vi "GCFS.vi"() -> ()   [LabVIEW 2024]
uses:
  DataCluster_GCFS.ctl
  <vilib>/userDefined/High Color/IMAQdx.ctl
  <vilib>/vision/Image Controls.llb/IMAQ Image.ctl
  <vilib>/Platform/TimedLoop/XDataNode/timing_clust.ctl
  <vilib>/Platform/TimedLoop/XDataNode/nitl_modes.ctl
  <vilib>/Platform/TimedLoop/XDataNode/wakeup.ctl
  af9ea1de-6e94-45bd-9990-e3be68a33346.vi
  <vilib>/addons/_JKI Toolkits/State Machine/_JKI_lib_State_Machine.llb/Select State(s)_err__jki_lib_state_machine.vi
  <extravilib>/ChannelInstances/Tag-t'DataCluster_GCFS.ctl'/Read With Abort.vi
  <extravilib>/ChannelInstances/Stream-c(t'IMAQ Image.ctl',str,a[.,.](str),a[.,.](str),bool)/Read With Abort.vi
  <extravilib>/ChannelInstances/Stream-c(t'IMAQ Image.ctl',str,a[.,.](str),a[.,.](str),bool)/Write With Abort.vi
  <extravilib>/ChannelInstances/Tag-t'DataCluster_GCFS.ctl'/Write With Abort.vi
  <extravilib>/ChannelInstances/Stream-c(t'IMAQ Image.ctl',str,a[.,.](str),a[.,.](str),bool)/EndpointRead.vi
  <extravilib>/ChannelInstances/Stream-c(t'IMAQ Image.ctl',str,a[.,.](str),a[.,.](str),bool)/Endpoint.vi
  <extravilib>/ChannelInstances/Stream-c(t'IMAQ Image.ctl',str,a[.,.](str),a[.,.](str),bool)/Instantiate.vi
  <extravilib>/ChannelInstances/Tag-t'DataCluster_GCFS.ctl'/Instantiate.vi
  <extravilib>/ChannelInstances/Tag-t'DataCluster_GCFS.ctl'/EndpointRead.vi
  <extravilib>/ChannelInstances/Stream-c(t'IMAQ Image.ctl',str,a[.,.](str),a[.,.](str),bool)/)Channel.vi
  <resource>/ChannelSupport/_ChannelSupport/WaitIfNeeded.vi
  <vilib>/addons/_JKI Toolkits/State Machine/_JKI_lib_State_Machine.llb/Periodic Trigger__ogtk__JKI-SM__jki_lib_state_machine.vi
  <vilib>/Utility/file.llb/Write Delimited Spreadsheet (DBL).vi
  <extravilib>/ChannelInstances/Tag-t'DataCluster_GCFS.ctl'/Endpoint.vi
  <vilib>/platform/TimedLoop/XDataNode/XDataNode.xnode
  <vilib>/regexp/Match Regular Expression.xnode
  <vilib>/vision/driver/NI_Vision_Acquisition_Software.lvlib
  <extravilib>/ChannelInstances/Tag-t'DataCluster_GCFS.ctl'.lvlib
  <vilib>/Platform/TimedLoop/XDataNode/XDNodeRunTimeDep.lvlib
  <extravilib>/ChannelInstances/Stream-c(t'IMAQ Image.ctl',str,a[.,.](str),a[.,.](str),bool).lvlib
panel:
  in  "Use Test Image":bool
  out "Save loop":i32
  out "Data Loop":i32
  out "Temperature":dbl
  in  "Freezing value":sgl=250.0
  in  "OFF":bool
  in  "Cool":bool
  in  "Heat":bool
  in  "Get Image":bool
  out "Frezz Image":T1(plugin-control)
  out "Droplet binary":T1(plugin-control)
  out "Droplet Position":T1(plugin-control)
  out "Grap Image":T1(plugin-control)
  in  "Active":bool
  in  "Sample name":string
  in  "Grap Position Image":bool
  out "Statusstring":string
  out "Particle Measurements (Pixels) (Particle Analysis 1)":dbl[][](array[numeric]) format="%.2f"
  out "Number of Particles":i32
  in  "Exit":bool
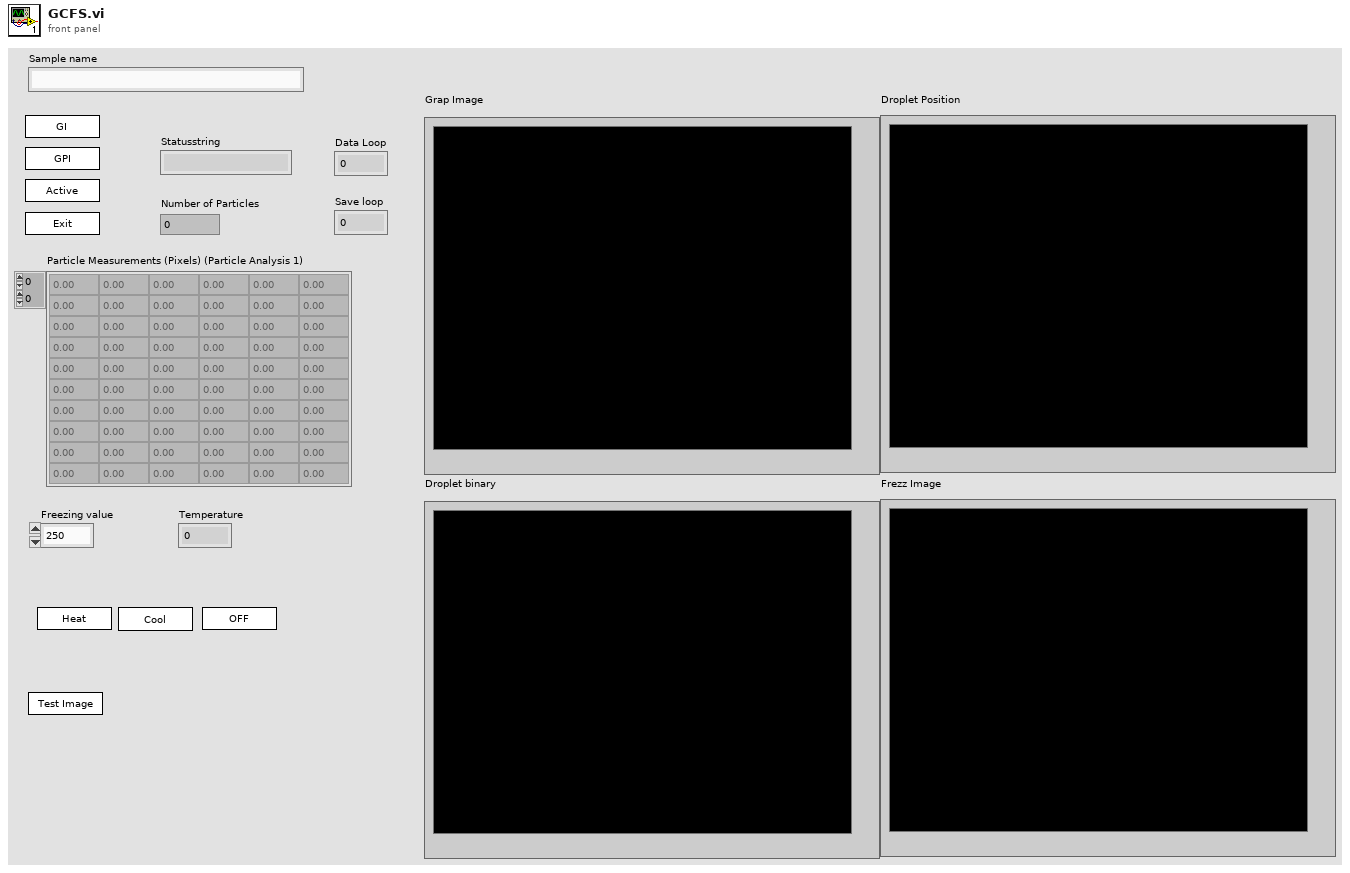
[diagram p1: front panel]
types:
  T1 = typedef "IMAQ Image.ctl" = refnum<image>
  T2 = typedef "DataCluster_GCFS.ctl" = cluster{"Core":cluster{"Current VI Reference":refnum<vi>, "Close Panel on Exit?":bool}, "Your Boolean data":bool, "Your string data":string, "Camera Cluster":cluster{"Session":T3, "Image":T1, "Position Image":T1, "PixelVal Image":T1, "Position Image Binary":T1, "Lable Image":T1}, "Data In Cluster":cluster{"Images":cluster{"Position Image path":path, "Sample folder path":path, "Label Image path":path}, "Sample Name":string, "Sample Rate":i32, "Gradient Buffer":i32, "Data Acquisition.Setup.TempGrad":dbl, "Control.PID gains":cluster{"proportional gain (Kc)":dbl, "integral time (Ti, min)":dbl, "derivative time (Td, min)":dbl}}, "Active":bool, "Ready":bool, "Exit":bool, "Arduino":cluster{"Connection":bool, "Port":refnum<visa-resource-name>, "State":string}, "Program_Start":string, "Data Out Cluster":cluster{"Particle Measurements (Pixels) (Particle Analysis 1)":dbl[][], "Number of droplets":i32, "PosImg_Timestamp":string}, "PSU":cluster{"Connection":bool, "Port":refnum<visa-resource-name>, "State":string}}
  T3 = typedef "IMAQdx.ctl" = refnum<k21>
  T4 = enum32{"Invalid", "Standard", "Closed", "Hidden", "Minimized", "Maximized"}
  T5 = enum32{"invalid app kind", "Development System", "Run Time System", "Student Edition", "Embedded LabVIEW", "Evaluation", "Custom"}
  T6 = cluster{"Desired Font (Application)":enum16{"User-specified Font", "Application Font", "System Font", "Dialog Font"}, "[User-specified Font]":cluster{"Font Name":string, "Size":i16, "Strikeout?":bool, "Italic?":bool, "Underline?":bool, "Outline?":bool, "Shadow?":bool, "Bold?":bool, "Rotation Angle":dbl}, "Horizontal Alignment":i16, "Vertical Alignment":i16}
  T7 = cluster{"Current VI Reference":refnum<vi>, "Close Panel on Exit?":bool}
  T8 = typedef "Image Type" = u32
  T9 = cluster{"Type":u32, "Version":u32, "Flags":u32, "SerialNumberHigh":u32, "SerialNumberLow":u32, "BusType":u32, "InterfaceName":string, "VendorName":string, "ModelName":string, "CameraFileName":string, "CameraAttributeURL":string}[]
  T10 = typedef "Tag-t'DataCluster_GCFS.ctl'.lvlib/))Channel.ctl" = refnum<queue>
  T11 = cluster{"Image To Save":T1, "Snap timestamp":string, "Pixel values":string[][], "Freezing points":string[][], "FreezingData":bool}
  T12 = typedef "XDNodeRunTimeDep.lvlib/timing_clust.ctl" = cluster{"Expected End [f-1]":u64, "Actual End [f-1]":u64, "Finished Late? [f-1]":bool, "Expected End [i-1]":u64, "Actual End [i-1]":u64, "Finished Late? [i-1]":bool, "Expected Start [i]":u64, "Actual Start [i]":u64, "Expected Start [f]":u64, "Actual Start [f]":u64, "Source Name":string, "Structure Name":string, "Period":i64, "Deadline":i64, "Offset":i64, "Start":i64, "Priority":i32, "Timeout":i32, "Mode":T13, "Wakeup Reason":T14, "Error":errorcluster, "Source Type":string, "Secondary Source Type":string, "Global End Time":u64, "Global Start Time":u64, "Frame Duration":u64, "Iteration Duration":u64, "Assigned CPU":i32, "I/O Scan Engine Mode":u32}
  T13 = typedef "XDNodeRunTimeDep.lvlib/nitl_modes.ctl" = enum32{"No Change", "Process missed periods, maintain original phase", "Discard missed periods, maintain original phase", "Process missed periods, ignore original phase", "Discard missed periods, ignore original phase"}
  T14 = typedef "XDNodeRunTimeDep.lvlib/wakeup.ctl" = enum32{"Normal", "Aborted", "Asynchronous wakeup", "Timing source error", "Timed loop error", "Timeout"}
  T15 = typedef "Stream-c(t'IMAQ Image.ctl',str,a[.,.](str),a[.,.](str),bool).lvlib/)Channel.ctl" = refnum<queue>
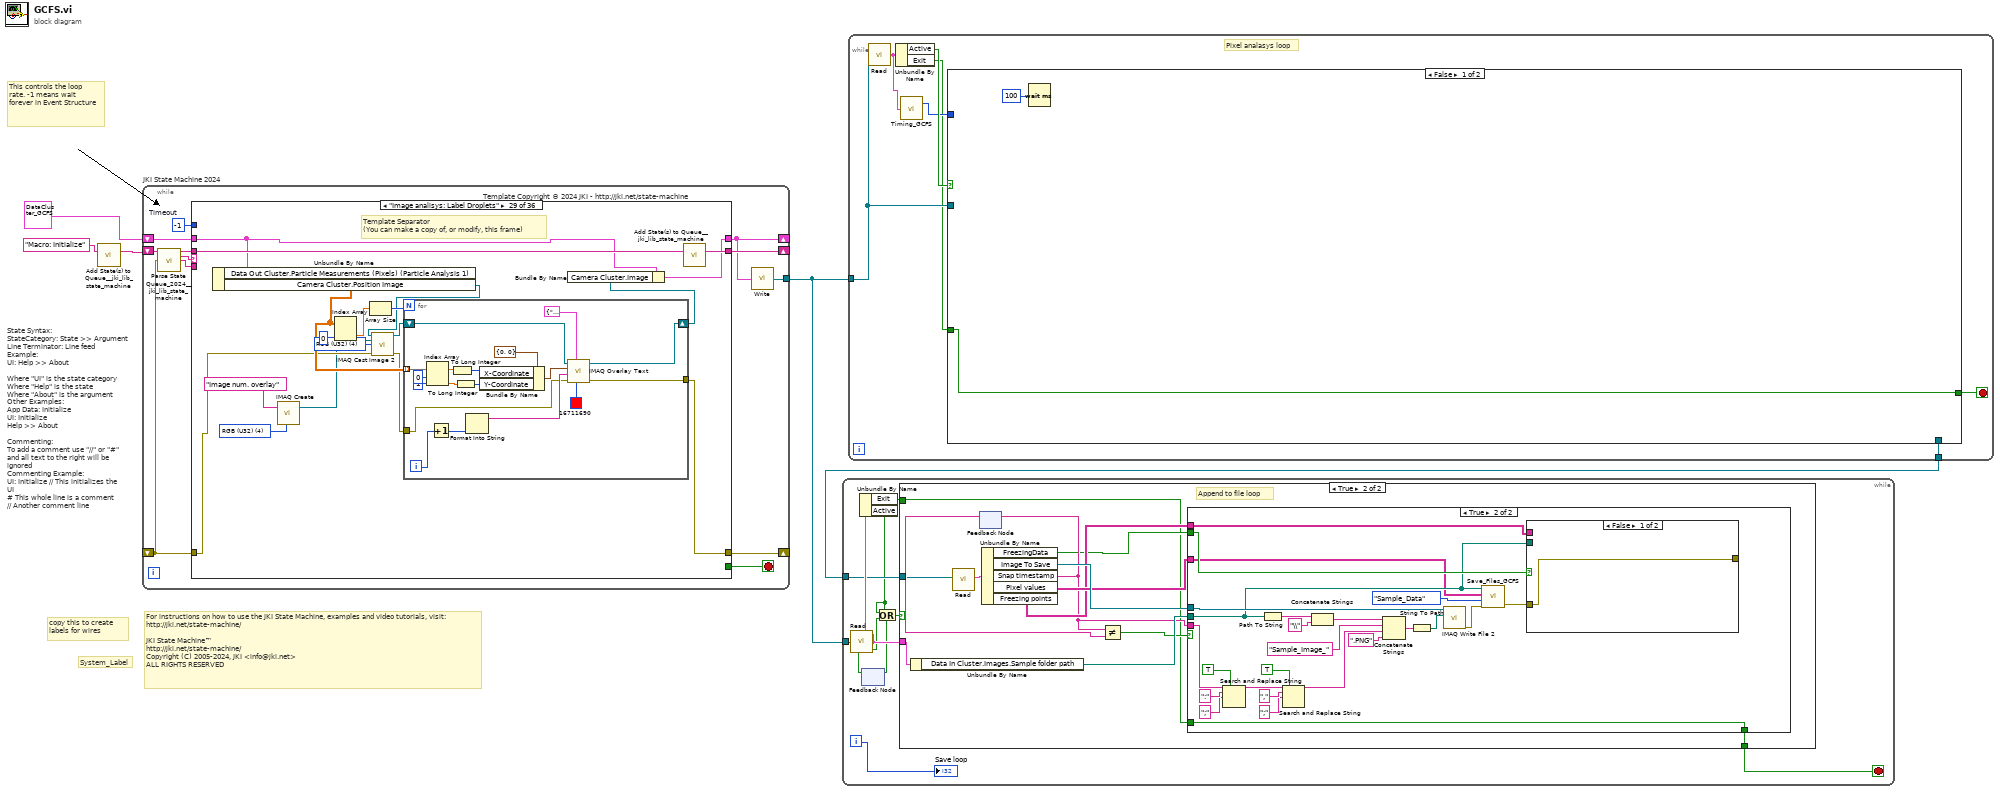
[diagram p0: block diagram]
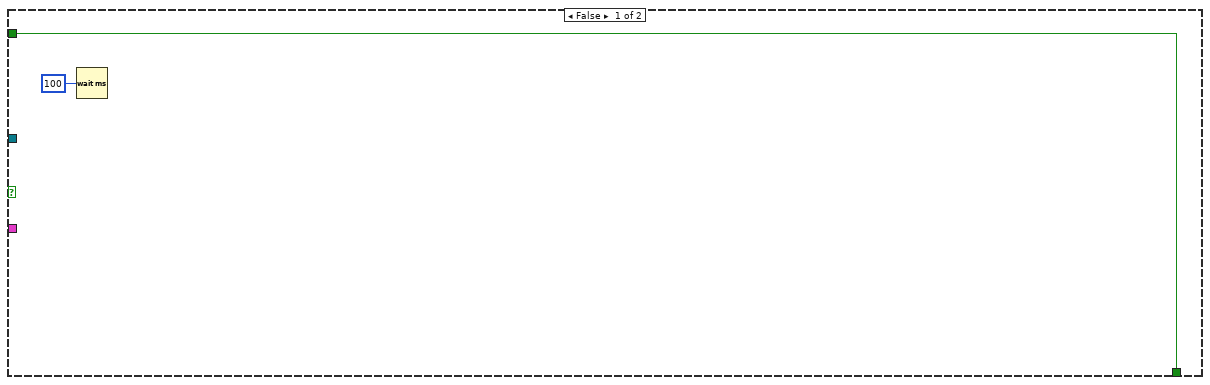
[diagram p2: hidden frame]
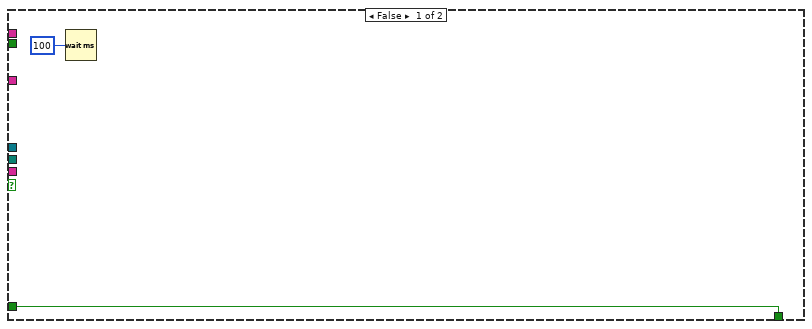
[diagram p3: hidden frame]
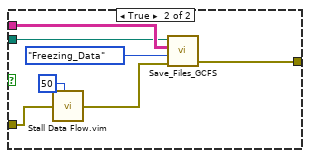
[diagram p4: hidden frame]
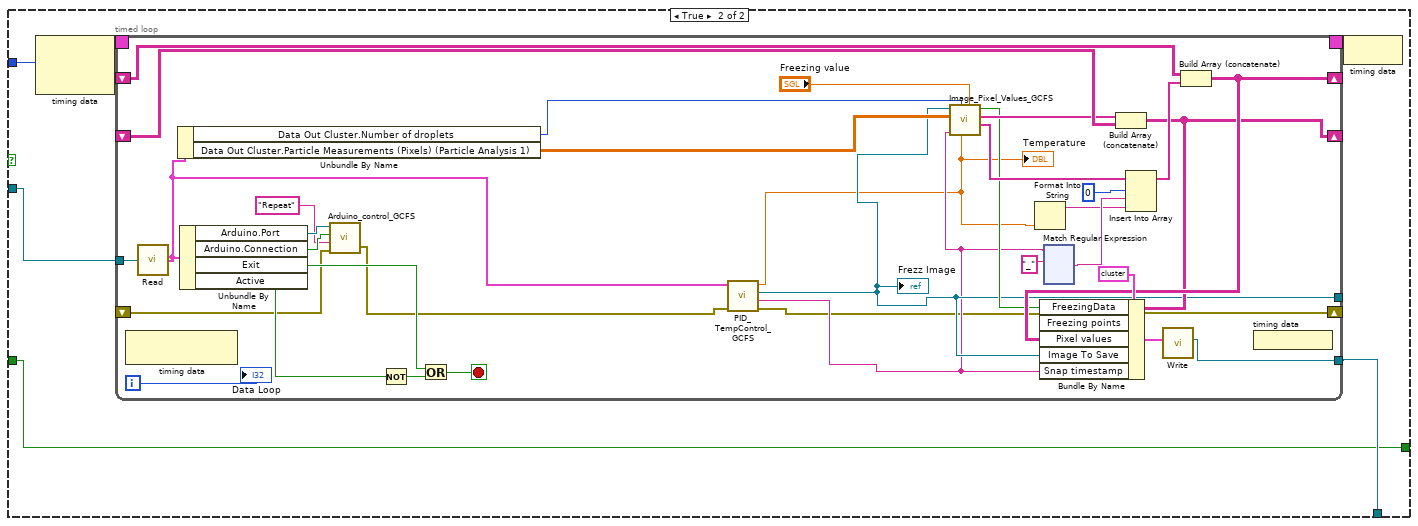
[diagram p5: hidden frame]
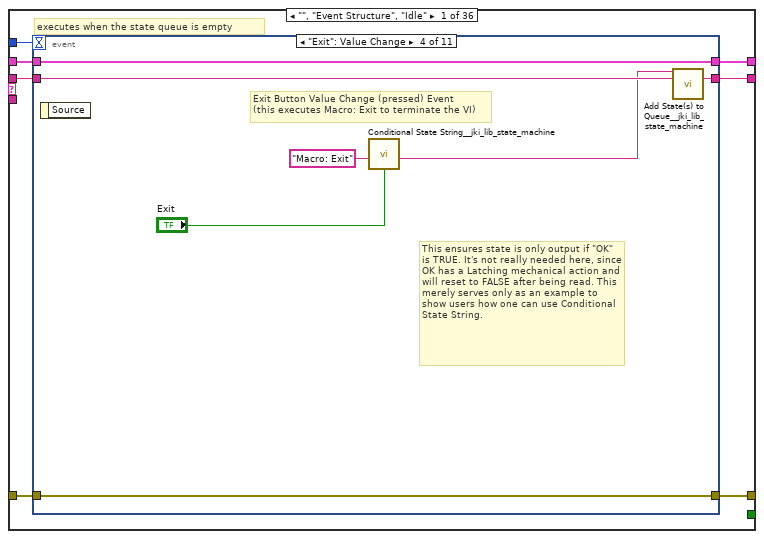
[diagram p6: hidden frame]
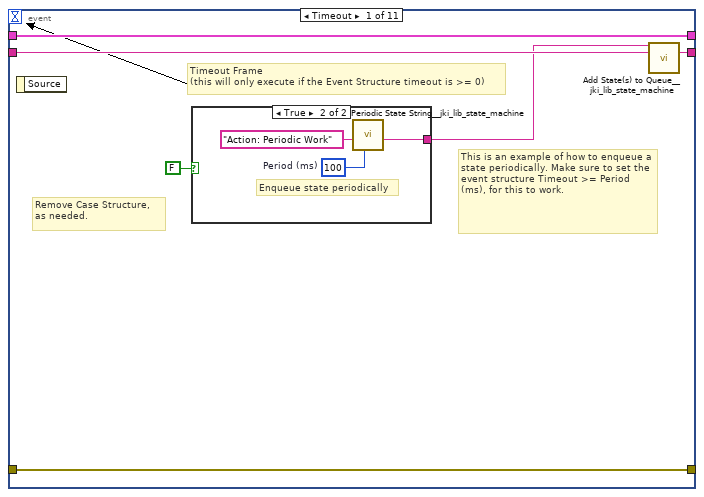
[diagram p7: hidden frame]
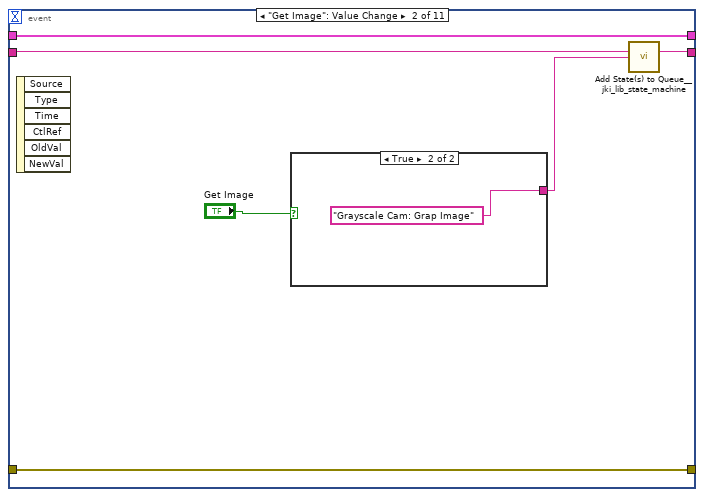
[diagram p9: hidden frame]
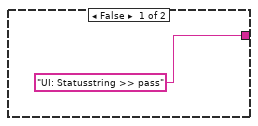
[diagram p10: hidden frame]
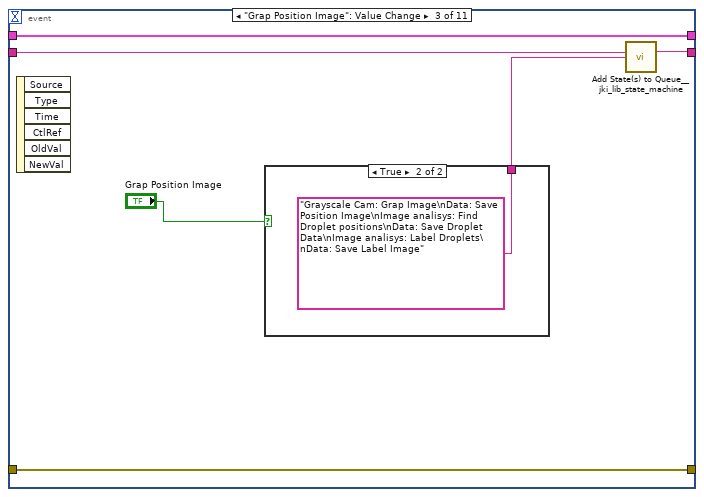
[diagram p11: hidden frame]
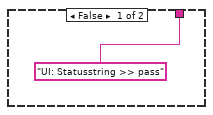
[diagram p12: hidden frame]
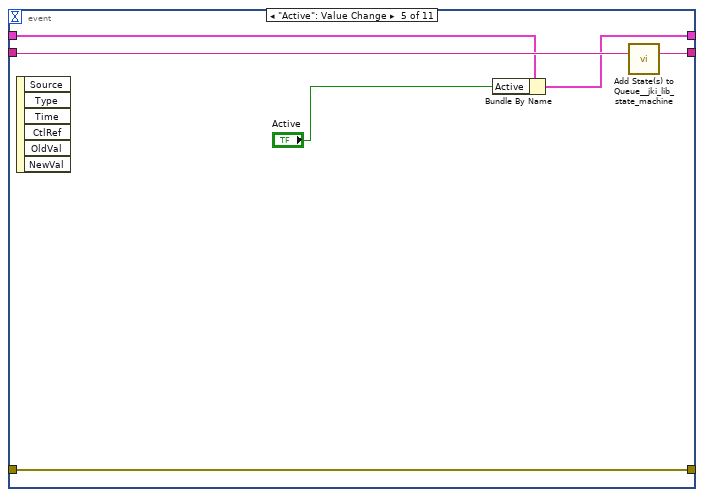
[diagram p13: hidden frame]
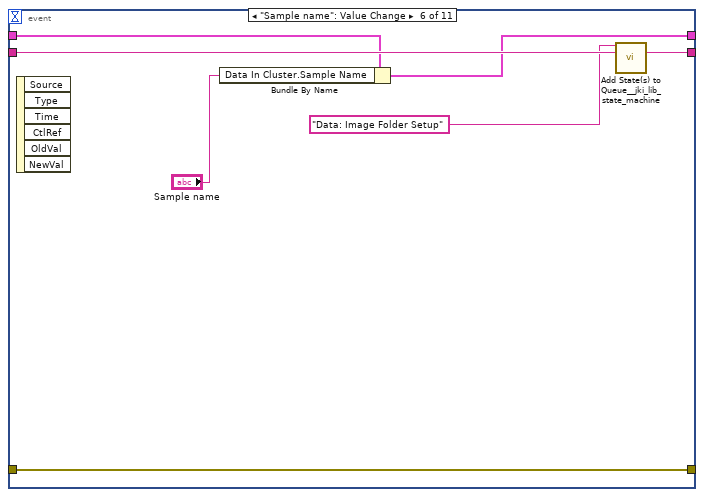
[diagram p14: hidden frame]
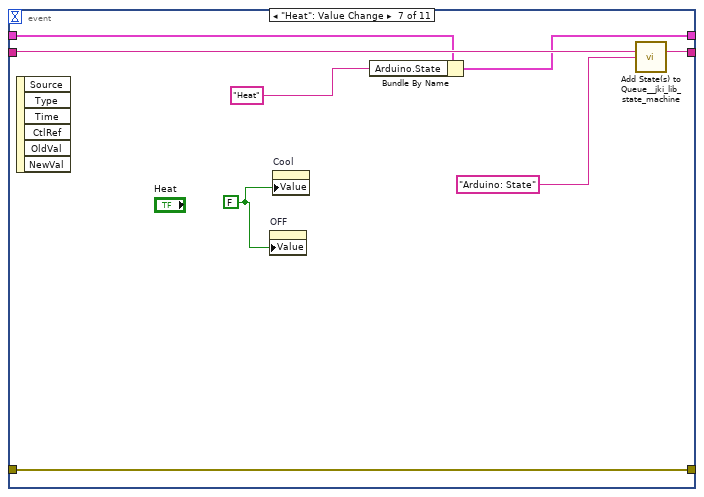
[diagram p15: hidden frame]
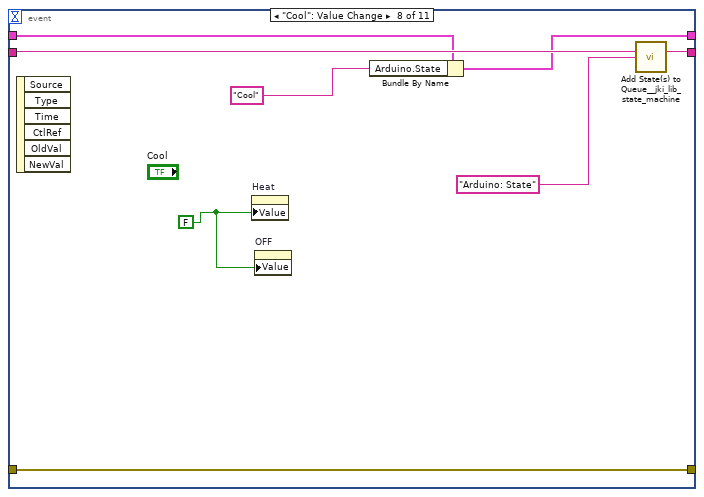
[diagram p16: hidden frame]
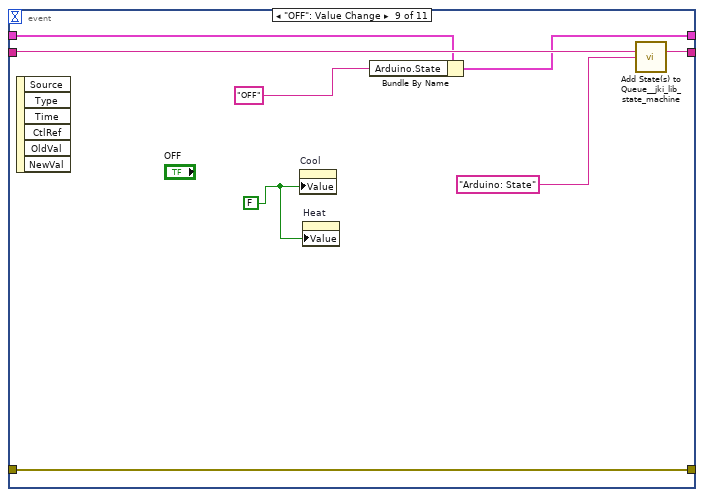
[diagram p17: hidden frame]
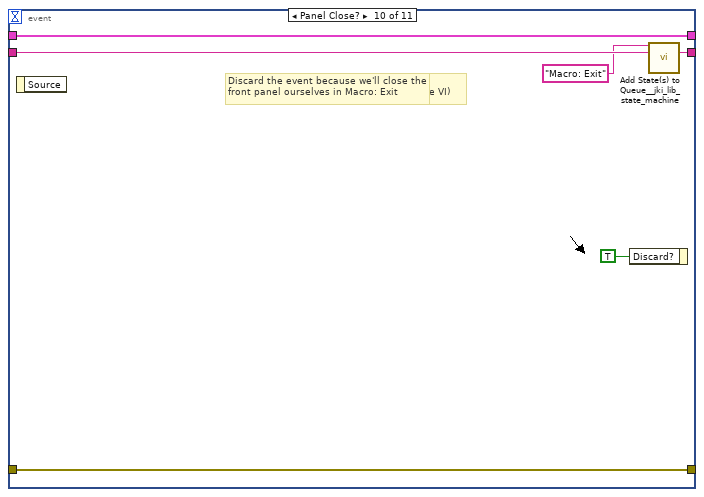
[diagram p18: hidden frame]
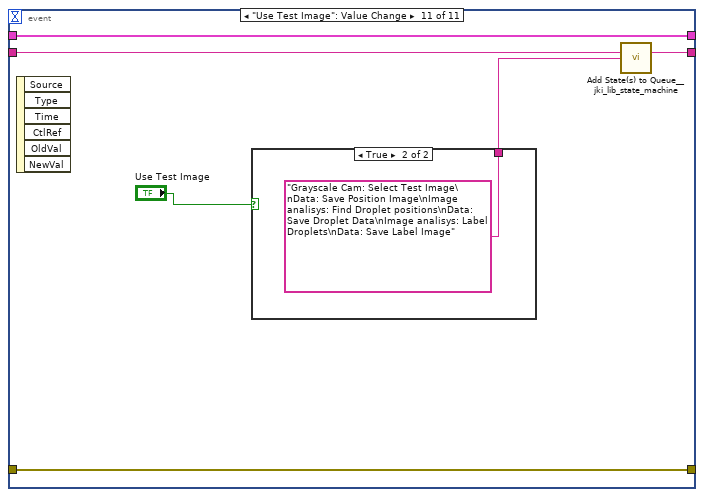
[diagram p19: hidden frame]
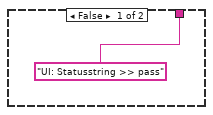
[diagram p20: hidden frame]
diagram:
  # "For instructions on how to use the JKI State Machine, examples and video tutorials, visit:\nhttp://jki.net/state-machine/\n\nJKI State Machine™\nhttp://jki.net/state-machine/\nCopyright (C) 2005-2024, JKI <info@jki.net>\nALL RIGHTS RESERVED"
  # "State Syntax:\nStateCategory: State >> Argument\nLine Terminator: Line feed\nExample:\nUI: Help >> About\n\nWhere \"UI\" is the state category\nWhere \"Help\" is the state\nWhere \"About\" is the argument\nOther Examples:\nApp Data: Initialize\nUI: Initialize\nHelp >> About\n\nCommenting:\nTo add a comment use \"//\" or \"#\" and all text to the right will be ignored\nCommenting Example:\nUI: Initialize // This initializes the UI\n# This whole line is a comment\n// Another comment line"
  # "copy this to create labels for wires"
  # "This controls the loop rate. -1 means wait forever in Event Structure"
  # "System_Label"
  n1 = call <vilib>:"Add State(s) to Queue__jki_lib_state_machine.vi"("State(s) in (\"\")"="Macro: Initialize") -> ("States Out"=w5:string)  [unwired: 14 in]
  n2 = while "JKI State Machine 2024" {
    shift-right: [w10] -> _
    shift-left: T2 {"Core"={"Current VI Reference"=refnum, "Close Panel on Exit?"=FALSE}, "Your Boolean data"=FALSE, "Your string data"="", "Camera Cluster"={"Session"="", "Image"=refnum, "Position Image"=refnum, "PixelVal Image"=refnum, "Position Image Binary"=refnum, "Lable Image"=refnum}, "Data In Cluster"={"Images"={"Position Image path"=path "", "Sample folder path"=path "", "Label Image path"=path ""}, "Sample Name"="", "Sample Rate"=0, "Gradient Buffer"=0, "Data Acquisition.Setup.TempGrad"=0.0, "Control.PID gains"={"proportional gain (Kc)"=0.0, "integral time (Ti, min)"=0.0, "derivative time (Td, min)"=0.0}}, "Active"=FALSE, "Ready"=FALSE, "Exit"=FALSE, "Arduino"={"Connection"=FALSE, "Port"="", "State"=""}, "Program_Start"="", "Data Out Cluster"={"Particle Measurements (Pixels) (Particle Analysis 1)"=[], "Number of droplets"=0, "PosImg_Timestamp"=""}, "PSU"={"Connection"=FALSE, "Port"="", "State"=""}} -> [w9]
    shift-right: [w13] -> _
    shift-left: _ -> [w7]
    shift-right: [w12] -> _
    shift-left: w5 -> [w14]
    tunnel: [w6] -> w2
    stop <- w11 stop-if-true
    w8 = -1  # Timeout
    # "Template Copyright © 2024 JKI - http://jki.net/state-machine"
    n3 = call <vilib>:"Parse State Queue_2024__jki_lib_state_machine.vi"("State Queue"=w14, "Error In (no error)"=w7) -> ("Remaining States"=w16:string, "Current State"=w17:string, "Arguments"=w15:string)  [unwired: 11 in]
    n4 = case shown="\"Image analisys: Label Droplets\"" w17 {
      selector: w17 -> [_ _ w112 _ _ _ _ _ _ _ _ _ _ _ _ _ _ _ _ _ _ _ _ _ _ _ _ _ _ _ _ _ _ _ _ _]
      tunnel: w16 -> [w24 w111 w116 w135 w145 w156 w160 w165 w174 w178 w189 w195 w215 w237 w253 w270 w274 w293 w297 w303 w314 w384 w388 w401 w426 w451 w455 w465 w483 w505 w513 w523 w531 w543 w550 w557]
      tunnel: w15 -> [_ _ _ _ w140 _ _ _ _ _ _ _ _ _ _ _ _ _ _ w298 w308 w380 _ _ _ _ _ _ _ _ _ _ _ _ _ _]
      tunnel: w9 -> [w22 w108 w114 w128 w142 w152 w157 w162 w172 w175 w185 w190 w202 w226 w242 w268 w271 w291 w295 w301 w310 w381 w385 w392 w417 w445 w452 w460 w477 w502 w509 w519 w527 w540 w548 w551]
      tunnel: [w21 w109 w118 w132 errorcluster {"status"=FALSE, "code"=0, "source"=""} ("error out") w154 w158 w163 w169 w176 w187 w191 w204 w227 w243 w254 w272 w284 w294 w299 w311 w382 w386 w389 w419 w431 w453 w461 w467 w503 w510 w515 w525 w541 w545 w552] -> w13
      tunnel: w7 -> [w18 w109 w117 w132 w141 w154 w158 w163 w169 w176 w187 w192 w206 w228 w244 w255 w272 w286 w294 w300 w312 w382 w386 w393 w421 w438 w453 w462 w472 w503 w511 w516 w526 w541 w546 w553]
      tunnel: [w23 w110 w115 w134 w144 w155 w159 w164 w173 w177 w188 w194 w214 w236 w252 w269 w273 w292 w296 w302 w313 w383 w387 w400 w425 w450 w454 w464 w482 w504 w512 w522 w530 w542 w549 w556] -> w12
      tunnel: [_ _ _ _ _ TRUE _ _ _ _ _ _ _ _ _ _ _ _ _ _ _ _ _ _ _ _ _ _ _ _ _ _ _ _ _ _] -> w11
      tunnel: [w20 w108 w114 w133 w142 w151 w157 w162 w172 w175 w184 w190 w201 w225 w241 w268 w271 w291 w295 w301 w310 w381 w385 w391 w418 w449 w452 w459 w476 w502 w508 w518 w524 w540 w547 w551] -> w10
      tunnel: w8 -> [w19 _ _ _ _ _ _ _ _ _ _ _ _ _ _ _ _ _ _ _ _ _ _ _ _ _ _ _ _ _ _ _ _ _ _ _]
      frame "", "Event Structure", "Idle" {
        # "executes when the state queue is empty"
        n5 = event shown="[3] \"Exit\": Value Change" {
          selector: _ -> [_ _ _ _ _ _ _ _ _ _ _]
          dyn-events: _ -> [_ _ _ _ _ _ _ _ _ _ _]
          timeout: w19 -> [_ _ _ _ _ _ _ _ _ _ _]
          tunnel: w24 -> [w30 w36 w45 w56 w61 w68 w76 w84 w92 w99 w105]
          tunnel: [w29 w37 w46 w55 w62 w69 w77 w85 w93 w98 w104] -> w23
          tunnel: w22 -> [w27 w38 w47 w53 w60 w66 w73 w81 w89 w96 w103]
          tunnel: [w28 w39 w42 w54 w57 w63 w74 w82 w90 w97 w102] -> w21
          tunnel: w18 -> [w28 w39 w42 w54 w57 w63 w74 w82 w90 w97 w102]
          tunnel: [w27 w38 w47 w53 w59 w65 w72 w80 w88 w96 w103] -> w20
          event Timeout {
            # "Remove Case Structure, as needed."
            # "This is an example of how to enqueue a state periodically. Make sure to set the event structure Timeout >= Period (ms), for this to work."
            # "Timeout Frame\n(this will only execute if the Event Structure timeout is >= 0)"
            n6 = event-data() -> ()  [unwired: 1 in, 1 out]
            n7 = case shown="True" FALSE {
              tunnel: [_ w33] -> w26
              frame False {
              }
              frame True {
                w31 = u32 100  # Period (ms)
                # "Enqueue state periodically"
                n8 = call <vilib>:"Periodic State String__jki_lib_state_machine.vi"("Period (ms)"=w31, "State"="Action: Periodic Work") -> ("State Out"=w33:string)  [unwired: 9 in]
              }
            }
            n9 = call <vilib>:"Add State(s) to Queue__jki_lib_state_machine.vi"("State(s) in Front (\"\")"=w26, "State(s) in (\"\")"=w30) -> ("States Out"=w29:string)  [unwired: 13 in]
          }
          event "Get Image": Value Change {
            n10 = event-data() -> ()  [unwired: 1 in, 6 out]
            n11 = case shown="True" "Get Image" {
              tunnel: ["UI: Statusstring >> pass" "Grayscale Cam: Grap Image"] -> w35
              frame False {
              }
              frame True {
              }
            }
            n12 = call <vilib>:"Add State(s) to Queue__jki_lib_state_machine.vi"("State(s) in (\"\")"=w36, "State(s) at Back (\"\")"=w35) -> ("States Out"=w37:string)  [unwired: 13 in]
          }
          event "Grap Position Image": Value Change {
            n13 = event-data() -> ()  [unwired: 1 in, 6 out]
            n14 = case shown="True" "Grap Position Image" {
              tunnel: ["UI: Statusstring >> pass" "Grayscale Cam: Grap Image\nData: Save Position Image\nImage analisys: Find Droplet positions\nData: Save Droplet Data\nImage analisys: Label Droplets\nData: Save Label Image"] -> w43
              frame False {
              }
              frame True {
              }
            }
            n15 = call <vilib>:"Add State(s) to Queue__jki_lib_state_machine.vi"("State(s) in (\"\")"=w45, "State(s) at Back (\"\")"=w43) -> ("States Out"=w46:string)  [unwired: 13 in]
          }
          event "Exit": Value Change {
            # "This ensures state is only output if \"OK\" is TRUE. It's not really needed here, since OK has a Latching mechanical action and will reset to FALSE after being read. This merely serves only as an example to show users how one can use Conditional State String."
            # "Exit Button Value Change (pressed) Event\n(this executes Macro: Exit to terminate the VI)"
            n16 = event-data() -> ()  [unwired: 1 in, 1 out]
            n17 = call <vilib>:"Conditional State String__jki_lib_state_machine.vi"("Do State(s)?"="Exit", "State"="Macro: Exit") -> ("State Out"=w50:string)  [unwired: 7 in]
            n18 = call <vilib>:"Add State(s) to Queue__jki_lib_state_machine.vi"("State(s) in Front (\"\")"=w50, "State(s) in (\"\")"=w56) -> ("States Out"=w55:string)  [unwired: 13 in]
          }
          event "Active": Value Change {
            n19 = event-data() -> ()  [unwired: 1 in, 6 out]
            n20 = Bundle By Name(cluster=w60, "Active"="Active") -> (w59:T2)
            n21 = call <vilib>:"Add State(s) to Queue__jki_lib_state_machine.vi"("State(s) in (\"\")"=w61) -> ("States Out"=w62:string)  [unwired: 14 in]
          }
          event "Sample name": Value Change {
            n22 = event-data() -> ()  [unwired: 1 in, 6 out]
            n23 = Bundle By Name(cluster=w66, "Data In Cluster.Sample Name"="Sample name") -> (w65:T2)
            n24 = call <vilib>:"Add State(s) to Queue__jki_lib_state_machine.vi"("State(s) in Front (\"\")"="Data: Image Folder Setup", "State(s) in (\"\")"=w68) -> ("States Out"=w69:string)  [unwired: 13 in]
          }
          event "Heat": Value Change {
            w70 = FALSE
            n25 = event-data() -> ()  [unwired: 1 in, 6 out]
            n26 = property on="OFF" class="Bool (strict)"("Value"=w70) -> ()  [unwired: 2 in, 2 out]
            n27 = property on="Cool" class="Bool (strict)"("Value"=w70) -> ()  [unwired: 2 in, 2 out]
            n28 = Bundle By Name(cluster=w73, "Arduino.State"="Heat") -> (w72:T2)
            n29 = call <vilib>:"Add State(s) to Queue__jki_lib_state_machine.vi"("State(s) in (\"\")"=w76, "State(s) at Back (\"\")"="Arduino: State" ("State(s) at Back (\"\")")) -> ("States Out"=w77:string)  [unwired: 13 in]
          }
          event "Cool": Value Change {
            w78 = FALSE
            n30 = event-data() -> ()  [unwired: 1 in, 6 out]
            n31 = property on="Heat" class="Bool (strict)"("Value"=w78) -> ()  [unwired: 2 in, 2 out]
            n32 = property on="OFF" class="Bool (strict)"("Value"=w78) -> ()  [unwired: 2 in, 2 out]
            n33 = Bundle By Name(cluster=w81, "Arduino.State"="Cool") -> (w80:T2)
            n34 = call <vilib>:"Add State(s) to Queue__jki_lib_state_machine.vi"("State(s) in (\"\")"=w84, "State(s) at Back (\"\")"="Arduino: State" ("State(s) at Back (\"\")")) -> ("States Out"=w85:string)  [unwired: 13 in]
          }
          event "OFF": Value Change {
            w86 = FALSE
            n35 = event-data() -> ()  [unwired: 1 in, 6 out]
            n36 = property on="Cool" class="Bool (strict)"("Value"=w86) -> ()  [unwired: 2 in, 2 out]
            n37 = property on="Heat" class="Bool (strict)"("Value"=w86) -> ()  [unwired: 2 in, 2 out]
            n38 = Bundle By Name(cluster=w89, "Arduino.State"="OFF") -> (w88:T2)
            n39 = call <vilib>:"Add State(s) to Queue__jki_lib_state_machine.vi"("State(s) in (\"\")"=w92, "State(s) at Back (\"\")"="Arduino: State" ("State(s) at Back (\"\")")) -> ("States Out"=w93:string)  [unwired: 13 in]
          }
          event Panel Close? {
            # "Discard the event because we'll close the front panel ourselves in Macro: Exit"
            # "Close Panel button (pressed) Event\n(this executes Macro: Exit to terminate the VI)"
            n40 = event-data() -> ()  [unwired: 1 in, 1 out]
            n41 = event-data("Discard?"=TRUE) -> ()  [unwired: 1 in, 1 out]
            n42 = call <vilib>:"Add State(s) to Queue__jki_lib_state_machine.vi"("State(s) in Front (\"\")"="Macro: Exit", "State(s) in (\"\")"=w99) -> ("States Out"=w98:string)  [unwired: 13 in]
          }
          event "Use Test Image": Value Change {
            n43 = event-data() -> ()  [unwired: 1 in, 6 out]
            n44 = case shown="True" "Use Test Image" {
              tunnel: ["UI: Statusstring >> pass" "Grayscale Cam: Select Test Image\nData: Save Position Image\nImage analisys: Find Droplet positions\nData: Save Droplet Data\nImage analisys: Label Droplets\nData: Save Label Image"] -> w100
              frame False {
              }
              frame True {
              }
            }
            n45 = call <vilib>:"Add State(s) to Queue__jki_lib_state_machine.vi"("State(s) in (\"\")"=w105, "State(s) at Back (\"\")"=w100) -> ("States Out"=w104:string)  [unwired: 13 in]
          }
        }
      }
      frame "---------- Core ----------" {
        # "Do not put any code in this frame.\n(it is a separator no-op)"
        n46 = call <vilib>:"Add State(s) to Queue__jki_lib_state_machine.vi"("State(s) in (\"\")"=w111) -> ("States Out"=w110:string)  [unwired: 14 in]
      }
      frame Default {
        w121 = 42 items=["No error", "Argument error", "Memory is full", "Out of zone", "End of file", "File already open", "Generic file I/O error", "File not found", "File permission error", "Disk is full", "Duplicate path", "Too many files open", "System feature not enabled", "Resource file not found", "Cannot add resource", "Resource not found", "Image not found", "Image memory error", "Pen does not exist", "Config type invalid", "Config token not found", "Config parse error", "Config memory error", "Bad external code format", "Bad external code offset", "External code not present", "Null window", "Destroy window error", "Null menu", "Print aborted", "Bad print record", "Print driver error", "Windows error during printing", "Memory error during printing", "Print dialog error", "Generic print error", "Invalid device refnum", "Device not found", "Device parameter error", "Device unit error", "Cannot open device", "Device call aborted", "Generic error", "Cancelled by user", "Object ID too low", "Object ID too high", "Object not in heap", "Unknown heap", "Unknown object (invalid DefProc)", "Unknown object (DefProc not in table)", "Message out of range", "Invalid (null) method", "Unknown message", "Manager call not supported", "Bad address", "Network operation in progress", "Network operation timed out", "Connection is busy", "Network attribute not supported", "Network error", "Address in use", "System out of memory", "Connection aborted", "Connection refused", "Not connected", "Already connected", "Connection closed", "Initialization error (interapplication manager)", "Bad occurrence", "Wait on unbound occurrence handler", "Occurrence queue overflow", "Datalog type conflict", "Unused", "Unrecognized type (interapplication manager)", "Memory corrupt", "Failed to make temporary DLL", "Old CIN version", "Drag socket not found", "Failed to load drop-object", "Failed to register OLE object", "Failed to release OLE object", "Format specifier type mismatch", "Unknown format specifier", "Too few format specifiers", "Too many format specifiers", "Scan failed", "Newer CIN version", "Error converting to variant", "Runtime menu error", "Password tampered", "Variant attribute not found", "Incompatible variant data type", "Event data is not available", "Event Store is not present", "Occurrence is not found", "Event Queue is not created", "Event info is not available", "Refnum passed is NULL", "Error retrieving Class GUID", "Error retrieving CoClass GUID", "Error retrieving TypeLib GUID.", "Bad built application magic bytes.", "Specific driver is different from the specific driver associated with the Logical Name.", "There is no session opened to the class driver.", "Max Error", "MAX - Error with config objects", "MAX - Error loading configuration", "MAX - Group not supported"]
        # "Current State"
        # "Do not delete, rename, or modify this frame.\n(this is used to capture unhandled states and typos)"
        # "Handle mistyped state name (developer tool)"
        n47 = Format Into String(format string="Software Exception: Unhandled State \"%s\"." ("message"), error in=w117, w112) -> (resulting string=w120:string, error out=w119:errorcluster)  [unwired: 1 in]
        n48 = call <vilib>:"Error Cluster From Error Code.vi"("show call chain? (False)"=TRUE, "error in (no error)"=w119, "error message (\"\")"=w120, "error code (0)"=w121) -> ("error out"=w118:errorcluster)  [unwired: 5 in]
        n49 = call <vilib>:"Add State(s) to Queue__jki_lib_state_machine.vi"("State(s) in (\"\")"=w116) -> ("States Out"=w115:string)  [unwired: 14 in]
      }
      frame "Initialize Core Data" {
        # "Do not delete, rename, or modify this frame.\n(this is used to determine panel behavior on exit)"
        # "originally closed?"
        # "exe?"
        # "If panel starts closed or is an EXE, then close it when we exit"
        n50 = property class="VI"() -> ("FP.State"=w125:T4)  [unwired: 2 in, 2 out]
        n51 = property class="App"() -> ("App.Kind"=w131:T5)  [unwired: 2 in, 2 out]
        n52 = control-ref of="Current VI Reference"() -> (w126:refnum<vi>)
        n53 = Equal?(x=w125, y=T4."Closed" ("Front Panel Window:State")) -> (x = y?=w123:bool)
        n54 = Equal?(x=w131, y=T5."Run Time System" ("Application:Kind")) -> (x = y?=w129:bool)
        n55 = Or(x=w123, y=w129) -> (x .or. y?=w127:bool)
        n56 = Bundle By Name(cluster=w128, "Core.Current VI Reference"=w126, "Core.Close Panel on Exit?"=w127) -> (w133:T2)
        n57 = call <vilib>:"Add State(s) to Queue__jki_lib_state_machine.vi"("State(s) in (\"\")"=w135) -> ("States Out"=w134:string)  [unwired: 14 in]
      }
      frame "Error Handler" {
        # "When running as sourcecode, this function will add previous state data to the error message to aid the developer in troubleshoot errors.\nIf run as an executable, no additional information is added to the error message."
        # "This state receives both Errors and Warnings which is how the Status of this wire can be FALSE"
        # "Unhandled Error -- Display it"
        # "Handle any errors or warnings here.\nYou can also output any states to clean-up after errors or warnings occur"
        # "Clear error or warning"
        n58 = disable-structure shown="Default" {
          disable-tunnel: w141 -> [w148 w149]
          disable-tunnel: w140 -> [w147 _]
          disable-tunnel: [w146 w149] -> w139
          frame condition #0 (active) {
            n59 = call <vilib>:"Append Error Details__jki_lib_state_machine.vi"("error in (no error)"=w148, "Previous State and Argument(s)"=w147) -> ("error out"=w146:errorcluster)  [unwired: 9 in]
          }
          frame condition #1 {
          }
        }
        n60 = call <vilib>:"General Error Handler.vi"("error in (no error)"=w139) -> ()  [unwired: 10 in, 5 out]
        n61 = call-poly <vilib>:"Select State(s)__jki_lib_state_machine.vi"("State(s) if True (\"\")"="/* Post Error States", "Select"=w139, "State(s) if False (\"\")"="/* Post Warning States") -> ("States Out"=w137:string)  [unwired: 12 in]
        n62 = call <vilib>:"Add State(s) to Queue__jki_lib_state_machine.vi"("State(s) in Front (\"\")"=w137, "State(s) in (\"\")"=w145) -> ("States Out"=w144:string)  [unwired: 13 in]
      }
      frame "Exit" {
        # "Do not put any code in this frame.\n(No errors that occur here will be handled.)"
        n63 = Bundle By Name(cluster=w152, "Exit"=TRUE) -> (w151:T2)
        n64 = call <vilib>:"Add State(s) to Queue__jki_lib_state_machine.vi"("State(s) in (\"\")"=w156) -> ("States Out"=w155:string)  [unwired: 14 in]
      }
      frame "---------- Macro ----------" {
        # "Do not put any code in this frame.\n(It is a separator no-op. You can make a copy of this frame to create a new Macro frame)"
        n65 = call <vilib>:"Add State(s) to Queue__jki_lib_state_machine.vi"("State(s) in (\"\")"=w160) -> ("States Out"=w159:string)  [unwired: 14 in]
      }
      frame "Macro: Initialize" {
        w161 = "Data: Initialize\nInitialize Core Data\nUI: Statusstring >> Initialysing\nUI: Front Panel State >> Open\nUI: Initialize\nData: Image Folder Setup\nArduino: Initialize\nGrayscale Cam: Initialize\nPSU: Initialize\nUI: Statusstring >> Initialysation done\n"  # Data: Initialize Initialize Core Data UI: Statusstring >> Initialysing UI: Front Panel State >> Open UI: Initialize Data: Image Folder Setup Arduino: Initialize Grayscale Cam: Initialize PSU: Initialize UI: Statusstring >> Initialysation done
        # "Initialization Macro\n(This is called once, when the VI starts)"
        n66 = call <vilib>:"Add State(s) to Queue__jki_lib_state_machine.vi"("State(s) in Front (\"\")"=w161, "State(s) in (\"\")"=w165) -> ("States Out"=w164:string)  [unwired: 13 in]
      }
      frame "Macro: Exit" {
        # "Exit Macro\n(This is called once, when the VI exits)"
        n67 = Unbundle By Name(w172) -> ("Core.Close Panel on Exit?"=w167:bool)
        n68 = call <vilib>:"Conditional State String__jki_lib_state_machine.vi"("Do State(s)?"=w167, "State"="UI: Front Panel State >> Close") -> ("State Out"=w166:string)  [unwired: 7 in]
        n69 = call <vilib>:"Add State(s) to Queue__jki_lib_state_machine.vi"("State(s) in (\"\")"=w166, "State(s) at Back (\"\")"="UI: Uninitialize\nData: Cleanup\nExit") -> ("States Out"=w170:string)  [unwired: 13 in]
        n70 = call <vilib>:"Add State(s) to Queue__jki_lib_state_machine.vi"("State(s) in Front (\"\")"=w170, "State(s) in (\"\")"=w174) -> ("States Out"=w173:string)  [unwired: 13 in]
      }
      frame "---------- Data ----------" {
        # "Do not put any code in this frame.\n(It is a separator no-op. You can make a copy of this frame to create a new Data frame)"
        n71 = call <vilib>:"Add State(s) to Queue__jki_lib_state_machine.vi"("State(s) in (\"\")"=w178) -> ("States Out"=w177:string)  [unwired: 14 in]
      }
      frame "Data: Initialize" {
        w186 = T7 {"Current VI Reference"=refnum, "Close Panel on Exit?"=FALSE}  # Core
        # "do not delete - used by framework"
        # "Initialize the shift-register data, here.\n(data names are defined by what you wire into the bundle function)"
        n72 = local read "Sample name"() -> (w182:string)
        n73 = Equal?(x=w182, y="") -> (x = y?=w181:bool)
        n74 = call "Prompt User for Sample name"("Enable"=w181) -> ("Sample name"=w180:string)  [unwired: 16 in, 2 out]
        n75 = Select(t=w180, s=w181, f=w182) -> (s? t:f=w179:string)
        n76 = Bundle By Name(cluster=w185, "Core"=w186, "Data In Cluster.Sample Name"=w179) -> (w184:T2)
        n77 = local write "Sample name"(w179) -> ()
        n78 = call <vilib>:"Add State(s) to Queue__jki_lib_state_machine.vi"("State(s) in (\"\")"=w189) -> ("States Out"=w188:string)  [unwired: 14 in]
      }
      frame "Data: Cleanup" {
        # "Cleanup any data and references, here.\n(this is called automatically, by the Macro: Exit)"
        n79 = Unbundle By Name(w190) -> ("Core.Current VI Reference"=w193:refnum<vi>)
        n80 = Close Reference(reference=w193, error in (no error)=w192) -> (error out=w191:errorcluster)
        n81 = call <vilib>:"Add State(s) to Queue__jki_lib_state_machine.vi"("State(s) in (\"\")"=w195) -> ("States Out"=w194:string)  [unwired: 14 in]
      }
      frame "Data: Image Folder Setup" {
        w197 = "\\" ("string")
        # "Do not put any code in this frame.\n(It is a separator no-op. You can make a copy of this frame to create a new Data frame)"
        n82 = Unbundle By Name(w202) -> ("Data In Cluster.Sample Name"=w203:string)
        n83 = Format Date/Time String(time format string (%c)="%Y-%m-%d_%H;%M", UTC format=FALSE) -> (date/time string=w196:string)  [unwired: 1 in]
        n84 = call <vilib>:"Application Directory.vi"() -> ("Application Directory"=w212:path)
        n85 = Path To String(path=w212) -> (string=w211:string)
        n86 = Concatenate Strings(w211, w197, "Flat Surface Images" ("string"), w197, w203, w197, w196) -> (w209:string)
        n87 = String To Path(string=w209) -> (path=w210:path)
        n88 = call <vilib>:"Check if File or Folder Exists.vi"("error in (no error)"=w206, "path"=w210) -> ("error out"=w205:errorcluster, "file or folder exists?"=w208:bool, "dup path"=w207:path)  [unwired: 7 in]
        n89 = case shown="False" w208 {
          tunnel: w207 -> [w217 w221]
          tunnel: w205 -> [w219 w220]
          tunnel: [w218 w220] -> w204
          tunnel: [w216 w221] -> w200
          frame False {
            n90 = Create Folder(path (use dialog)=w217, error in=w219) -> (created path=w216:path, error out=w218:errorcluster)  [unwired: 1 in, 1 out]
          }
          frame True {
          }
        }
        n91 = Bundle By Name(cluster=w202, "Data In Cluster.Images.Sample folder path"=w200, "Program_Start"=w196) -> (w201:T2)
        n92 = call <vilib>:"Add State(s) to Queue__jki_lib_state_machine.vi"("State(s) in (\"\")"=w215) -> ("States Out"=w214:string)  [unwired: 14 in]
      }
      frame "Data: Save Position Image" {
        # "Do not put any code in this frame.\n(It is a separator no-op. You can make a copy of this frame to create a new Data frame)"
        n93 = Unbundle By Name(w226) -> ("Camera Cluster.Image"=w231:T1, "Data In Cluster.Images.Sample folder path"=w230:path, "Data Out Cluster.PosImg_Timestamp"=w229:string)
        n94 = Path To String(path=w230) -> (string=w232:string)
        n95 = Concatenate Strings(w232, "\\" ("string"), "Position_Image_" ("string"), w229, ".PNG" ("string")) -> (w235:string)
        n96 = String To Path(string=w235) -> (path=w224:path)
        n97 = call-poly "IMAQ Write File 2"("error in (no error)"=w228, "File Path"=w224, "Image"=w231) -> ("error out"=w227:errorcluster, "Image Out (duplicate)"=w222:T1)  [unwired: 7 in]
        "Droplet Position" <- w222
        n98 = Bundle By Name(cluster=w226, "Data In Cluster.Images.Position Image path"=w224, "Camera Cluster.Position Image"=w222) -> (w225:T2)
        n99 = call <vilib>:"Add State(s) to Queue__jki_lib_state_machine.vi"("State(s) in (\"\")"=w237) -> ("States Out"=w236:string)  [unwired: 14 in]
      }
      frame "Data: Save Label Image" {
        # "Do not put any code in this frame.\n(It is a separator no-op. You can make a copy of this frame to create a new Data frame)"
        n100 = Unbundle By Name(w242) -> ("Camera Cluster.Image"=w247:T1, "Data In Cluster.Images.Sample folder path"=w246:path, "Data Out Cluster.PosImg_Timestamp"=w245:string)
        n101 = Path To String(path=w246) -> (string=w248:string)
        n102 = Concatenate Strings(w248, "\\" ("string"), "Label_Image_" ("string"), w245, ".PNG" ("string")) -> (w251:string)
        n103 = String To Path(string=w251) -> (path=w240:path)
        n104 = call-poly "IMAQ Write File 2"("error in (no error)"=w244, "File Path"=w240, "Image"=w247) -> ("error out"=w243:errorcluster, "Image Out (duplicate)"=w238:T1)  [unwired: 7 in]
        n105 = Bundle By Name(cluster=w242, "Data In Cluster.Images.Label Image path"=w240, "Camera Cluster.Lable Image"=w238) -> (w241:T2)
        n106 = local write "Droplet Position"(w238) -> ()
        n107 = call <vilib>:"Add State(s) to Queue__jki_lib_state_machine.vi"("State(s) in (\"\")"=w253) -> ("States Out"=w252:string)  [unwired: 14 in]
      }
      frame "Data: Save Droplet Data" {
        # "Do not put any code in this frame.\n(It is a separator no-op. You can make a copy of this frame to create a new Data frame)"
        n108 = Unbundle By Name(w268) -> ("Data Out Cluster.Particle Measurements (Pixels) (Particle Analysis 1)"=w256:dbl[][], "Data In Cluster.Images.Sample folder path"=w267:path)
        n109 = Path To String(path=w267) -> (string=w261:string)
        n110 = Concatenate Strings(w261, "\\" ("string"), "Droplet_data" ("string"), ".csv" ("string")) -> (w266:string)
        n111 = String To Path(string=w266) -> (path=w259:path)
        n112 = call "DropletFile_Headers_GCFS.vi"("error in (no error)"=w255, "path"=w259) -> ("error out"=w257:errorcluster, "File path"=w258:path)
        n113 = call-poly <vilib>:"Write Delimited Spreadsheet.vi"("file path (dialog if empty)"=w258, "2D data"=w256, "append to file? (new file:F)"=TRUE, "error in (no error)"=w257, "delimiter (\\t)"=";" ("delimiter (\\t)")) -> ("error out"=w254:errorcluster)  [unwired: 9 in, 1 out]
        n114 = call <vilib>:"Add State(s) to Queue__jki_lib_state_machine.vi"("State(s) in (\"\")"=w270) -> ("States Out"=w269:string)  [unwired: 14 in]
      }
      frame "---------- UI ----------" {
        # "Do not put any code in this frame.\n(It is a separator no-op. You can make a copy of this frame to create a new UI frame)"
        n115 = call <vilib>:"Add State(s) to Queue__jki_lib_state_machine.vi"("State(s) in (\"\")"=w274) -> ("States Out"=w273:string)  [unwired: 14 in]
      }
      frame "UI: Initialize" {
        w276 = FALSE ("Cool")
        w280 = "\\" ("string")
        w288 = T8 6 items=["Grayscale (U8)", "Grayscale (I16)", "Grayscale (SGL)", "Complex (CSG)", "RGB (U32)", "HSL (U32)", "RGB (U64)", "Grayscale (U16)"] ("Image Type")
        w290 = T1 refnum ("Image")
        # "Initialize the User Interface, here.\n(this is called automatically, by the Macro: Initialize)"
        n116 = call <vilib>:"Application Directory.vi"() -> ("Application Directory"=w283:path)
        n117 = Path To String(path=w283) -> (string=w282:string)
        n118 = Concatenate Strings(w282, w280, "resources" ("string"), w280, "Logo_Full.png" ("string")) -> (w278:string)
        n119 = String To Path(string=w278) -> (path=w277:path)
        n120 = call "IMAQ Create"("Image Name"="Logo", "Image Type"=w288, "error in (no error)"=w286) -> ("New Image"=w287:T1, "error out"=w285:errorcluster)  [unwired: 2 in]
        n121 = property on="Cool" class="Bool (strict)"("Value"=w276) -> ()  [unwired: 2 in, 2 out]
        n122 = property on="OFF" class="Bool (strict)"("Value"=w276) -> ()  [unwired: 2 in, 2 out]
        n123 = call "IMAQ ReadFile 2"("File Path"=w277, "error in (no error)"=w285, "Image"=w287) -> ("error out"=w284:errorcluster)  [unwired: 4 in, 4 out]
        n124 = property on="Heat" class="Bool (strict)"("Value"=w276) -> ()  [unwired: 2 in, 2 out]
        n125 = property on="Active" class="Bool (strict)"("Value"=w276) -> ()  [unwired: 2 in, 2 out]
        n126 = property on="Particle Measurements (Pixels) (Particle Analysis 1)" class="Arr (strict)"("Value"=dbl[][] [] ("Particle Measurements (Pixels) (Particle Analysis 1)")) -> ()  [unwired: 2 in, 2 out]
        n127 = local write "Droplet binary"(w290) -> ()
        n128 = local write "Droplet Position"(w290) -> ()
        n129 = local write "Grap Image"(w290) -> ()
        n130 = local write "Frezz Image"(w290) -> ()
        n131 = call <vilib>:"Add State(s) to Queue__jki_lib_state_machine.vi"("State(s) in (\"\")"=w293) -> ("States Out"=w292:string)  [unwired: 14 in]
      }
      frame "UI: Uninitialize" {
        # "Cleanup the User Interface, here.\n(this is called automatically, by the Macro: Exit)"
        n132 = call <vilib>:"Add State(s) to Queue__jki_lib_state_machine.vi"("State(s) in (\"\")"=w297) -> ("States Out"=w296:string)  [unwired: 14 in]
      }
      frame "UI: Cursor Set" {
        # "Argument"
        # "Set and Unset Cursor Busy.\n(Usage: \"UI: Cursor Set >> Busy|Idle\")"
        n133 = case shown="\"Idle\", Default" w298 {
          tunnel: w300 -> [w305 w307]
          tunnel: [w304 w306] -> w299
          frame "Idle", Default {
            n134 = call <vilib>:"Unset Busy.vi"("error in (no error)"=w305) -> ("error out"=w304:errorcluster)  [unwired: 10 in]
          }
          frame "Busy" {
            n135 = call <vilib>:"Set Busy.vi"("error in (no error)"=w307) -> ("error out"=w306:errorcluster)  [unwired: 9 in, 1 out]
          }
        }
        n136 = call <vilib>:"Add State(s) to Queue__jki_lib_state_machine.vi"("State(s) in (\"\")"=w303) -> ("States Out"=w302:string)  [unwired: 14 in]
      }
      frame "UI: Front Panel State" {
        # "Argument"
        # "Set Front Panel Open or Closed\n(Usage: \"UI: Front Panel State >> Open|Close\")"
        n137 = Unbundle By Name(w310) -> ("Core.Current VI Reference"=w309:refnum<vi>)
        n138 = case shown="\"Open\", \"Standard\", Default" w308 {
          tunnel: w312 -> [w320 w335 w346 w359 w372]
          tunnel: [w322 w336 w348 w361 w374] -> w311
          tunnel: w309 -> [w321 w333 w347 w360 w373]
          frame "Open", "Standard", Default {
            w315 = T4."Standard" ("State")
            n139 = property class="VI"(reference=w321, error in=w320) -> (reference out=w318:refnum<vi>, error out=w319:errorcluster, "FP.State"=w317:T4)
            n140 = Not Equal?(x=w317, y=w315) -> (x != y?=w316:bool)
            n141 = case shown="True" w316 {
              tunnel: [w326 w328] -> w322
              tunnel: w319 -> [w325 w328]
              tunnel: w318 -> [w324 _]
              tunnel: w315 -> [w323 _]
              frame True {
                n142 = invoke class="VI" method="FP.Open"(reference=w324, error in=w325, "Activate"=TRUE, "State"=w323) -> (error out=w326:errorcluster)  [unwired: 1 in, 4 out]
              }
              frame False {
              }
            }
          }
          frame "Close", "Closed" {
            n143 = property class="VI"(reference=w333, error in=w335) -> (reference out=w332:refnum<vi>, error out=w334:errorcluster, "FP.State"=w330:T4)
            n144 = Not Equal?(x=w330, y=T4."Closed" ("Front Panel Window:State")) -> (x != y?=w329:bool)
            n145 = case shown="True" w329 {
              tunnel: [w337 w340] -> w336
              tunnel: w334 -> [w337 w339]
              tunnel: w332 -> [_ w338]
              frame False {
              }
              frame True {
                n146 = invoke class="VI" method="FP.Close"(reference=w338, error in=w339) -> (error out=w340:errorcluster)  [unwired: 1 in, 2 out]
              }
            }
          }
          frame "Hidden", "Hide" {
            w341 = T4."Hidden" ("State")
            n147 = property class="VI"(reference=w347, error in=w346) -> (reference out=w344:refnum<vi>, error out=w345:errorcluster, "FP.State"=w343:T4)
            n148 = Not Equal?(x=w343, y=w341) -> (x != y?=w342:bool)
            n149 = case shown="True" w342 {
              tunnel: [w352 w353] -> w348
              tunnel: w345 -> [w351 w353]
              tunnel: w344 -> [w350 _]
              tunnel: w341 -> [w349 _]
              frame True {
                n150 = invoke class="VI" method="FP.Open"(reference=w350, error in=w351, "State"=w349) -> (error out=w352:errorcluster)  [unwired: 2 in, 4 out]
              }
              frame False {
              }
            }
          }
          frame "Minimize", "Minimized" {
            w354 = T4."Minimized" ("State")
            n151 = property class="VI"(reference=w360, error in=w359) -> (reference out=w357:refnum<vi>, error out=w358:errorcluster, "FP.State"=w356:T4)
            n152 = Not Equal?(x=w356, y=w354) -> (x != y?=w355:bool)
            n153 = case shown="True" w355 {
              tunnel: [w365 w366] -> w361
              tunnel: w358 -> [w364 w366]
              tunnel: w357 -> [w363 _]
              tunnel: w354 -> [w362 _]
              frame True {
                n154 = invoke class="VI" method="FP.Open"(reference=w363, error in=w364, "State"=w362) -> (error out=w365:errorcluster)  [unwired: 2 in, 4 out]
              }
              frame False {
              }
            }
          }
          frame "Maximize", "Maximized" {
            w367 = T4."Maximized" ("State")
            n155 = property class="VI"(reference=w373, error in=w372) -> (reference out=w370:refnum<vi>, error out=w371:errorcluster, "FP.State"=w369:T4)
            n156 = Not Equal?(x=w369, y=w367) -> (x != y?=w368:bool)
            n157 = case shown="True" w368 {
              tunnel: [w378 w379] -> w374
              tunnel: w371 -> [w377 w379]
              tunnel: w370 -> [w376 _]
              tunnel: w367 -> [w375 _]
              frame True {
                n158 = invoke class="VI" method="FP.Open"(reference=w376, error in=w377, "State"=w375) -> (error out=w378:errorcluster)  [unwired: 2 in, 4 out]
              }
              frame False {
              }
            }
          }
        }
        n159 = call <vilib>:"Add State(s) to Queue__jki_lib_state_machine.vi"("State(s) in (\"\")"=w314) -> ("States Out"=w313:string)  [unwired: 14 in]
      }
      frame "UI: Statusstring" {
        # "Do not put any code in this frame.\n(It is a separator no-op. You can make a copy of this frame to create a new UI frame)"
        n160 = call <vilib>:"Add State(s) to Queue__jki_lib_state_machine.vi"("State(s) in (\"\")"=w384) -> ("States Out"=w383:string)  [unwired: 14 in]
        "Statusstring" <- w380
      }
      frame "---------- Grayscale Cam ----------" {
        # "Template Separator\n(You can make a copy of, or modify, this frame)"
        n161 = call <vilib>:"Add State(s) to Queue__jki_lib_state_machine.vi"("State(s) in (\"\")"=w388) -> ("States Out"=w387:string)  [unwired: 14 in]
      }
      frame "Grayscale Cam: Initialize" {
        # "Template Separator\n(You can make a copy of, or modify, this frame)"
        n162 = call <vilib>:"IMAQdx Enumerate Cameras.vi"("error in"=w393) -> ("error out"=w394:errorcluster, "Camera Information Array"=w398:T9)  [unwired: 9 in]
        n163 = Array Size(array=w398) -> (size(s)=w399:i32)
        n164 = for {
          N: w399 -> [_]
          tunnel: w398 -> [w409] mode=indexing
          shift-right: [w407] -> w397
          shift-left: _ -> [w402]
          n165 = Unbundle By Name(w409) -> ("InterfaceName"=w408:string, "VendorName"=w406:string)
          n166 = Match True/False String(2:"" ("false string"), 3:"JAI" ("true string"), 4:w406) -> (0:w403:bool)  [unwired: 1 out]
          n167 = Select(t=w408, s=w403, f=w402) -> (s? t:f=w407:string)
        }
        n168 = call <vilib>:"IMAQdx Open Camera.vi"("error in"=w394, "Session In"=w397) -> ("error out"=w396:errorcluster, "Session Out"=w395:T3)  [unwired: 8 in]
        n169 = call <vilib>:"IMAQdx Configure Grab.vi"("error in"=w396, "Session In"=w395) -> ("error out"=w389:errorcluster, "Session Out"=w390:T3)  [unwired: 8 in]
        n170 = Bundle By Name(cluster=w392, "Camera Cluster.Session"=w390) -> (w391:T2)
        n171 = call <vilib>:"Add State(s) to Queue__jki_lib_state_machine.vi"("State(s) in (\"\")"=w401) -> ("States Out"=w400:string)  [unwired: 14 in]
      }
      frame "Grayscale Cam: Grap Image" {
        w423 = T8 0 items=["Grayscale (U8)", "Grayscale (I16)", "Grayscale (SGL)", "Complex (CSG)", "RGB (U32)", "HSL (U32)", "RGB (U64)", "Grayscale (U16)"] ("Image Type")
        # "Template Separator\n(You can make a copy of, or modify, this frame)"
        n172 = Unbundle By Name(w417) -> ("Camera Cluster.Session"=w416:T3)
        n173 = call "IMAQ Create"("Image Name"="Image", "Image Type"=w423, "error in (no error)"=w421) -> ("New Image"=w422:T1, "error out"=w420:errorcluster)  [unwired: 2 in]
        n174 = Format Date/Time String(time format string (%c)="%Y-%m-%d_%H;%M;%S%3u", UTC format=FALSE) -> (date/time string=w411:string)  [unwired: 1 in]
        n175 = call <vilib>:"IMAQdx Grab2.vi"("Timeout (ms)"=5000, "error in"=w420, "Image In"=w422, "Session In"=w416) -> ("error out"=w419:errorcluster, "Image Out"=w410:T1, "Session Out"=w415:T3)  [unwired: 4 in, 1 out]
        "Grap Image" <- w410
        n176 = Bundle By Name(cluster=w417, "Camera Cluster.Session"=w415, "Camera Cluster.Image"=w410, "Data Out Cluster.PosImg_Timestamp"=w411) -> (w418:T2)
        n177 = call <vilib>:"Add State(s) to Queue__jki_lib_state_machine.vi"("State(s) in (\"\")"=w426) -> ("States Out"=w425:string)  [unwired: 14 in]
      }
      frame "Grayscale Cam: Select Test Image" {
        w435 = T8 0 items=["Grayscale (U8)", "Grayscale (I16)", "Grayscale (SGL)", "Complex (CSG)", "RGB (U32)", "HSL (U32)", "RGB (U64)", "Grayscale (U16)"] ("Image Type")
        w440 = "\\" ("string")
        # "Template Separator\n(You can make a copy of, or modify, this frame)"
        n178 = call <vilib>:"Application Directory.vi"() -> ("Application Directory"=w443:path)
        n179 = Path To String(path=w443) -> (string=w442:string)
        n180 = Concatenate Strings(w442, w440, "Flat Surface Images" ("string"), w440) -> (w441:string)
        n181 = String To Path(string=w441) -> (path=w439:path)
        n182 = call "File Dialog"("start path"=w439, "error in"=w438, "pattern (all files)"="*.png*") -> ("selected path"=w437:path, "error out"=w433:errorcluster)  [unwired: 9 in, 2 out]
        n183 = call "IMAQ Create"("Image Name"="Test", "Image Type"=w435, "error in (no error)"=w433) -> ("New Image"=w434:T1, "error out"=w432:errorcluster)  [unwired: 2 in]
        n184 = Format Date/Time String(time format string (%c)="%Y-%m-%d_%H;%M;%S%3u", UTC format=FALSE) -> (date/time string=w429:string)  [unwired: 1 in]
        n185 = call "IMAQ ReadFile 2"("File Path"=w437, "error in (no error)"=w432, "Image"=w434) -> ("error out"=w431:errorcluster, "Image Out"=w430:T1)  [unwired: 4 in, 3 out]
        n186 = Concatenate Strings("TEST_" ("string"), w429) -> (w427:string)
        n187 = Bundle By Name(cluster=w445, "Camera Cluster.Image"=w430, "Data Out Cluster.PosImg_Timestamp"=w427) -> (w449:T2)
        n188 = local write "Grap Image"(w430) -> ()
        n189 = call <vilib>:"Add State(s) to Queue__jki_lib_state_machine.vi"("State(s) in (\"\")"=w451) -> ("States Out"=w450:string)  [unwired: 14 in]
      }
      frame "---------- Image analisys ----------" {
        # "Template Separator\n(You can make a copy of, or modify, this frame)"
        n190 = call <vilib>:"Add State(s) to Queue__jki_lib_state_machine.vi"("State(s) in (\"\")"=w455) -> ("States Out"=w454:string)  [unwired: 14 in]
      }
      frame "Image analisys: Find Droplet positions" {
        # "Your code here.\n(You can make a copy of, or modify, this frame)"
        n191 = Unbundle By Name(w460) -> ("Camera Cluster.Position Image"=w463:T1)
        n192 = call "Vision Assistant"("Image In"=w463, "error in"=w462) -> ("Image Out"=w456:T1, "Number of Particles (Particle Analysis 1)"=w458:i32, "Particle Measurements (Pixels) (Particle Analysis 1)"=w457:dbl[][], "error out"=w461:errorcluster)  [unwired: 20 in, 2 out]
        "Number of Particles" <- w458
        "Particle Measurements (Pixels) (Particle Analysis 1)" <- w457
        "Droplet binary" <- w456
        n193 = Bundle By Name(cluster=w460, "Camera Cluster.Position Image Binary"=w456, "Data Out Cluster.Particle Measurements (Pixels) (Particle Analysis 1)"=w457, "Data Out Cluster.Number of droplets"=w458) -> (w459:T2)
        n194 = call <vilib>:"Add State(s) to Queue__jki_lib_state_machine.vi"("State(s) in (\"\")"=w465) -> ("States Out"=w464:string)  [unwired: 14 in]
      }
      frame "Image analisys: Label Droplets" {
        w468 = T8 4 items=["Grayscale (U8)", "Grayscale (I16)", "Grayscale (SGL)", "Complex (CSG)", "RGB (U32)", "HSL (U32)", "RGB (U64)", "Grayscale (U16)"] ("Image Type")
        w474 = T8 4 items=["Grayscale (U8)", "Grayscale (I16)", "Grayscale (SGL)", "Complex (CSG)", "RGB (U32)", "HSL (U32)", "RGB (U64)", "Grayscale (U16)"] ("Image Type")
        # "Template Separator\n(You can make a copy of, or modify, this frame)"
        n195 = Unbundle By Name(w477) -> ("Data Out Cluster.Particle Measurements (Pixels) (Particle Analysis 1)"=w478:dbl[][], "Camera Cluster.Position Image"=w475:T1)
        n196 = call "IMAQ Create"("Image Name"="Image num. overlay", "Image Type"=w468) -> ("New Image"=w470:T1)  [unwired: 3 in, 1 out]
        n197 = Index Array(array=w478, index (col)=0 ("disabled index (col)")) -> (element=w479:dbl[])  [unwired: 1 in]
        n198 = Array Size(array=w479) -> (size(s)=w480:i32)
        n199 = call "IMAQ Cast Image 2"("Image Src"=w475, "Image Dst"=w470, "Image Type"=w474, "error in (no error)"=w472) -> ("Image Dst Out"=w473:T1, "error out"=w471:errorcluster)  [unwired: 10 in]
        n200 = for {
          N: w480 -> [_]
          tunnel: w471 -> [w488]
          shift-right: [w498] -> w466
          shift-left: w473 -> [w499]
          tunnel: w478 -> [w497] mode=indexing
          tunnel: [w484] -> w467
          i -> [w487]
          n201 = Index Array(array=w497, index #1=0 ("index"), index #2=1 ("index")) -> (element #1=w492:dbl, element #2=w489:dbl)
          n202 = Increment(x=w487) -> (x+1=w486:i32)
          n203 = To Long Integer(number=w492) -> (32bit integer=w491:i32)
          n204 = To Long Integer(number=w489) -> (32bit integer=w490:i32)
          n205 = Format Into String(w486) -> (resulting string=w501:string)  [unwired: 3 in, 1 out]
          n206 = Bundle By Name(cluster=cluster{"X-Coordinate":i32, "Y-Coordinate":i32} {"X-Coordinate"=0, "Y-Coordinate"=0}, "X-Coordinate"=w491, "Y-Coordinate"=w490) -> (w493:cluster{"X-Coordinate":i32, "Y-Coordinate":i32})
          n207 = call "IMAQ Overlay Text"("Text Color (black)"=u32 16711690, "Font, Size & Style"=T6 {"Desired Font (Application)"=enum."Application Font", "[User-specified Font]"={"Font Name"="", "Size"=2, "Strikeout?"=FALSE, "Italic?"=FALSE, "Underline?"=FALSE, "Outline?"=FALSE, "Shadow?"=FALSE, "Bold?"=FALSE, "Rotation Angle"=0.0}, "Horizontal Alignment"=0, "Vertical Alignment"=0}, "error in (no error)"=w488, "String"=w501, "Origin"=w493, "Image"=w499) -> ("error out"=w484:errorcluster, "Image Out"=w498:T1)  [unwired: 4 in]
        }
        n208 = Bundle By Name(cluster=w477, "Camera Cluster.Image"=w466) -> (w476:T2)
        n209 = call <vilib>:"Add State(s) to Queue__jki_lib_state_machine.vi"("State(s) in (\"\")"=w483) -> ("States Out"=w482:string)  [unwired: 14 in]
      }
      frame "---------- Arduino ----------" {
        # "Template Separator\n(You can make a copy of, or modify, this frame)"
        n210 = call <vilib>:"Add State(s) to Queue__jki_lib_state_machine.vi"("State(s) in (\"\")"=w505) -> ("States Out"=w504:string)  [unwired: 14 in]
      }
      frame "Arduino: Initialize" {
        # "Template Separator\n(You can make a copy of, or modify, this frame)"
        n211 = call "Arduino_Initialization_GCFS.vi"("error in"=w511) -> ("error out"=w510:errorcluster, "Connection"=w506:bool, "VISA Arduino"=w507:refnum<visa-resource-name>)  [unwired: 7 in]
        n212 = Bundle By Name(cluster=w509, "Arduino.Port"=w507, "Arduino.Connection"=w506) -> (w508:T2)
        n213 = call <vilib>:"Add State(s) to Queue__jki_lib_state_machine.vi"("State(s) in (\"\")"=w513) -> ("States Out"=w512:string)  [unwired: 14 in]
      }
      frame "Arduino: State" {
        # "Template Separator\n(You can make a copy of, or modify, this frame)"
        n214 = Unbundle By Name(w519) -> ("Arduino.Port"=w521:refnum<visa-resource-name>, "Arduino.Connection"=w520:bool, "Arduino.State"=w514:string)
        n215 = call "Arduino_control_GCFS.vi"("error in (no error)"=w516, "Arguments"=w514, "Connection"=w520, "Port"=w521) -> ("error out"=w515:errorcluster, "Connection"=w517:bool)
        n216 = Bundle By Name(cluster=w519, "Arduino.Connection"=w517) -> (w518:T2)
        n217 = call <vilib>:"Add State(s) to Queue__jki_lib_state_machine.vi"("State(s) in (\"\")"=w523) -> ("States Out"=w522:string)  [unwired: 14 in]
      }
      frame "Arduino: Terminate" {
        # "Template Separator\n(You can make a copy of, or modify, this frame)"
        n218 = Unbundle By Name(w527) -> ("Arduino.Port"=w528:refnum<visa-resource-name>, "Arduino.Connection"=w529:bool)
        n219 = case shown="True" w529 {
          tunnel: w528 -> [_ w534]
          tunnel: w527 -> [w533 w539]
          tunnel: [w533 w537] -> w524
          tunnel: [w532 w536] -> w525
          tunnel: w526 -> [w532 w535]
          frame False {
          }
          frame True {
            w538 = FALSE ("Connections.Arduino.Connected")
            n220 = VISA Close(VISA resource name=w534, error in (no error)=w535) -> (error out=w536:errorcluster)
            n221 = Bundle By Name(cluster=w539, "Arduino.Connection"=w538, "Active"=w538) -> (w537:T2)
          }
        }
        n222 = call <vilib>:"Add State(s) to Queue__jki_lib_state_machine.vi"("State(s) in (\"\")"=w531) -> ("States Out"=w530:string)  [unwired: 14 in]
      }
      frame "---------- PSU ----------" {
        # "Template Separator\n(You can make a copy of, or modify, this frame)"
        n223 = call <vilib>:"Add State(s) to Queue__jki_lib_state_machine.vi"("State(s) in (\"\")"=w543) -> ("States Out"=w542:string)  [unwired: 14 in]
      }
      frame "PSU: Initialize" {
        # "Template Separator\n(You can make a copy of, or modify, this frame)"
        n224 = call "Connect_PSU_GCFS.vi"("error in (no error)"=w546, 5:w548) -> ("error out"=w545:errorcluster, "State out"=w544:string, "output cluster"=w547:T2)  [unwired: 1 in]
        n225 = call <vilib>:"Add State(s) to Queue__jki_lib_state_machine.vi"("State(s) in Front (\"\")"=w544, "State(s) in (\"\")"=w550) -> ("States Out"=w549:string)  [unwired: 13 in]
      }
      frame "PSU: Terminate" {
        # "Template Separator\n(You can make a copy of, or modify, this frame)"
        n226 = Unbundle By Name(w551) -> ("PSU.Port"=w554:refnum<visa-resource-name>, "PSU.Connection"=w555:bool)
        n227 = case shown="True" w555 {
          tunnel: w554 -> [_ w562]
          tunnel: w551 -> [w559 w565]
          tunnel: [w559 w563] -> _
          tunnel: [w558 w561] -> w552
          tunnel: w553 -> [w558 w560]
          frame False {
          }
          frame True {
            n228 = VISA Close(VISA resource name=w562, error in (no error)=w560) -> (error out=w561:errorcluster)
            n229 = Bundle By Name(cluster=w565, "PSU.Connection"=FALSE ("Connections.cDAQ.Connected")) -> (w563:T2)
          }
        }
        n230 = call <vilib>:"Add State(s) to Queue__jki_lib_state_machine.vi"("State(s) in (\"\")"=w557) -> ("States Out"=w556:string)  [unwired: 14 in]
      }
    }
    n231 = call <extravilib>:"Write.vi"("element"=w10) -> ("channel"=w6:T10)  [unwired: 1 out]
  }
  n232 = while {
    tunnel: w2 -> [w572]
    tunnel: [w570] -> w1
    stop <- w566 stop-if-true
    # "Pixel analasys loop"
    n233 = call <extravilib>:"Read.vi"("channel"=w572) -> ("element"=w568:T2)  [unwired: 1 in, 1 out]
    n234 = Unbundle By Name(w568) -> ("Active"=w571:bool, "Exit"=w567:bool)
    n235 = call "Timing_GCFS.vi"(0:w568) -> ("Sample dt (ms)"=w569:i64)  [unwired: 1 out]
    n236 = case shown="False" w571 {
      tunnel: w572 -> [_ w580]
      tunnel: w569 -> [_ w577]
      tunnel: [_ w576] -> w570
      tunnel: w567 -> [w573 w575]
      tunnel: [w573 w575] -> w566
      frame False {
        n237 = Wait (ms)(milliseconds to wait=u32 100) -> ()  [unwired: 1 out]
      }
      frame True {
        n238 = node-c288(w577) -> (w579:T12)  [unwired: 1 in]
        n239 = timed-loop {
          tunnel: w580 -> [w614]
          shift-right: [w584] -> _
          shift-left: _ -> [w599]
          timing: w579 -> [_]
          timing-out: [_] -> w578
          tunnel: [w586] -> _
          shift-right: [w606] -> _
          shift-left: _ -> [w607]
          tunnel: [w589] -> w576
          shift-right: [w602] -> _
          shift-left: _ -> [w603]
          i -> [w581]
          stop <- w590 stop-if-true
          n240 = node-c288() -> ()  [unwired: 1 in, 1 out]
          n241 = call <extravilib>:"Read.vi"("channel"=w614) -> ("element"=w588:T2)  [unwired: 1 in, 1 out]
          n242 = Unbundle By Name(w588) -> ("Data Out Cluster.Number of droplets"=w597:i32, "Data Out Cluster.Particle Measurements (Pixels) (Particle Analysis 1)"=w593:dbl[][])
          n243 = Unbundle By Name(w588) -> ("Arduino.Port"=w601:refnum<visa-resource-name>, "Arduino.Connection"=w600:bool, "Exit"=w611:bool, "Active"=w612:bool)
          n244 = call "Arduino_control_GCFS.vi"("error in (no error)"=w599, "Arguments"="Repeat", "Connection"=w600, "Port"=w601) -> ("error out"=w587:errorcluster)  [unwired: 1 out]
          n245 = Not(x=w612) -> (.not. x?=w613:bool)
          n246 = Or(x=w611, y=w613) -> (x .or. y?=w590:bool)
          n247 = call "PID_TempControl_GCFS.vi"("error in"=w587, 11:w588) -> ("error out"=w584:errorcluster, "date/time string"=w585:string, "Image Out"=w586:T1, "Temperature"=w583:dbl)  [unwired: 3 in, 3 out]
          "Frezz Image" <- w586
          "Temperature" <- w583
          n248 = call "Image_Pixel_Values_GCFS.vi"("Freezing value"="Freezing value", "Temperature"=w583, "Numeric"=w597, "date/time string"=w585, "Particle messurments"=w593, "Image in"=w586) -> ("Value_Array"=w594:string[], "Freezing_points"=w595:string[], "Freezing data"=w591:bool)  [unwired: 3 in]
          n249 = Format Into String(w583) -> (resulting string=w582:string)  [unwired: 3 in, 1 out]
          n250 = xnode "Match Regular Expression"("input string"=w585, "regular expression"="_" ("search string/char (-)")) -> ("after match"=w604:string)  [unwired: 4 in, 4 out]
          n251 = Build Array (concatenate)(w595, w603) -> (w602:string[][])
          n252 = Insert Into Array(array=w594, index=0, new element #1=w604, new element #2=w582) -> (w608:string[])
          n253 = Build Array (concatenate)(w607, w608) -> (w606:string[][])
          n254 = Bundle By Name(cluster=T11 {"Image To Save"=refnum, "Snap timestamp"="", "Pixel values"=[], "Freezing points"=[], "FreezingData"=FALSE}, "FreezingData"=w591, "Freezing points"=w602, "Pixel values"=w606, "Image To Save"=w586, "Snap timestamp"=w585) -> (w592:T11)
          n255 = call <extravilib>:"Write.vi"("element"=w592) -> ("channel"=w589:T15)  [unwired: 8 in, 2 out]
          n256 = node-c288() -> ()  [unwired: 1 out]
          "Data Loop" <- w581
        }
        n257 = node-c288(w578) -> ()
      }
    }
  }
  n258 = while {
    tunnel: w2 -> [w746]
    tunnel: w1 -> [w744]
    i -> [w741]
    stop <- w742 stop-if-true
    n259 = call <extravilib>:"Read.vi"("channel"=w746) -> ("element"=w745:T2)  [unwired: 1 in, 1 out]
    n260 = Unbundle By Name(w745) -> ("Exit"=w743:bool, "Active"=w739:bool)
    n261 = feedback-in #1(w739) -> ()
    n262 = feedback #1() -> (w738:bool)  [unwired: 1 in]
    n263 = Or(x=w739, y=w738) -> (x .or. y?=w740:bool)
    n264 = case shown="True" w740 {
      tunnel: w745 -> [_ w761]
      tunnel: w744 -> [_ w754]
      tunnel: w743 -> [w748 w750]
      tunnel: [w748 w749] -> w742
      frame False {
        n265 = Wait (ms)(milliseconds to wait=u32 100) -> ()  [unwired: 1 out]
      }
      frame True {
        # "Append to file loop"
        n266 = Unbundle By Name(w761) -> ("Data In Cluster.Images.Sample folder path"=w758:path)
        n267 = call <extravilib>:"Read.vi"("channel"=w754) -> ("element"=w753:T11)  [unwired: 6 in, 4 out]
        n268 = feedback #2() -> (w757:string)  [unwired: 1 in]
        n269 = Unbundle By Name(w753) -> ("FreezingData"=w752:bool, "Image To Save"=w760:T1, "Snap timestamp"=w755:string, "Pixel values"=w759:string[][], "Freezing points"=w756:string[][])
        n270 = feedback-in #2(w755) -> ()
        n271 = Not Equal?(x=w755, y=w757) -> (x != y?=w751:bool)
        n272 = case shown="True" w751 {
          tunnel: w758 -> [_ w767]
          tunnel: w760 -> [_ w784]
          tunnel: w759 -> [_ w765]
          tunnel: w756 -> [_ w768]
          tunnel: w755 -> [_ w781]
          tunnel: w752 -> [_ w769]
          tunnel: w750 -> [w762 w764]
          tunnel: [w762 w764] -> w749
          frame False {
            n273 = Wait (ms)(milliseconds to wait=u32 100) -> ()  [unwired: 1 out]
          }
          frame True {
            n274 = Search and Replace String(replace all?=TRUE ("replace all? (F)"), input string=w781, search string=":", replace string=";" ("replace string (\"\")")) -> (result string=w776:string)  [unwired: 4 in, 3 out]
            n275 = Path To String(path=w767) -> (string=w783:string)
            n276 = Search and Replace String(replace all?=TRUE ("replace all? (F)"), input string=w776, search string=",", replace string=";" ("replace string (\"\")")) -> (result string=w773:string)  [unwired: 4 in, 3 out]
            n277 = Concatenate Strings(w783, "\\" ("string")) -> (w782:string)
            n278 = Concatenate Strings(w782, "Sample_Image_" ("string"), w773, ".PNG" ("string")) -> (w788:string)
            n279 = String To Path(string=w788) -> (path=w786:path)
            n280 = call-poly "IMAQ Write File 2"("File Path"=w786, "Image"=w784) -> ("error out"=w771:errorcluster)  [unwired: 8 in, 1 out]
            n281 = call "Save_Files_GCFS.vi"("error in"=w771, "Enum"=enum16{"Freezing_Data", "Sample_Data"}."Sample_Data", "Array"=w765, "file path (use dialog)"=w767) -> ("error out"=w770:errorcluster)  [unwired: 1 in, 1 out]
            n282 = case shown="False" w769 {
              tunnel: w770 -> [w789 w792]
              tunnel: w768 -> [_ w795]
              tunnel: w767 -> [_ w794]
              tunnel: [w789 w793] -> _
              frame False {
              }
              frame True {
                n283 = call "Stall Data Flow.vim"("value in"=w792, "milliseconds to wait"=u32 50) -> ("value out"=w791:errorcluster)  [unwired: 1 out]
                n284 = call "Save_Files_GCFS.vi"("error in"=w791, "Enum"=enum16{"Freezing_Data", "Sample_Data"}."Freezing_Data", "Array"=w795, "file path (use dialog)"=w794) -> ("error out"=w793:errorcluster)  [unwired: 1 in, 1 out]
              }
            }
          }
        }
      }
    }
    "Save loop" <- w741
  }
